vi "filter_bad_values.vi"(11 "Array 3":i16[](array[numeric])) -> (3 "Array 4":i32[](array[numeric]))   [LabVIEW 2012]
uses:
  <vilib>/NXT/Dual Mode Library/prims/addArrayElements_int.vi
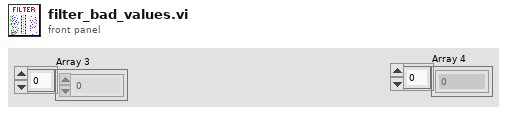
[diagram p1: front panel]
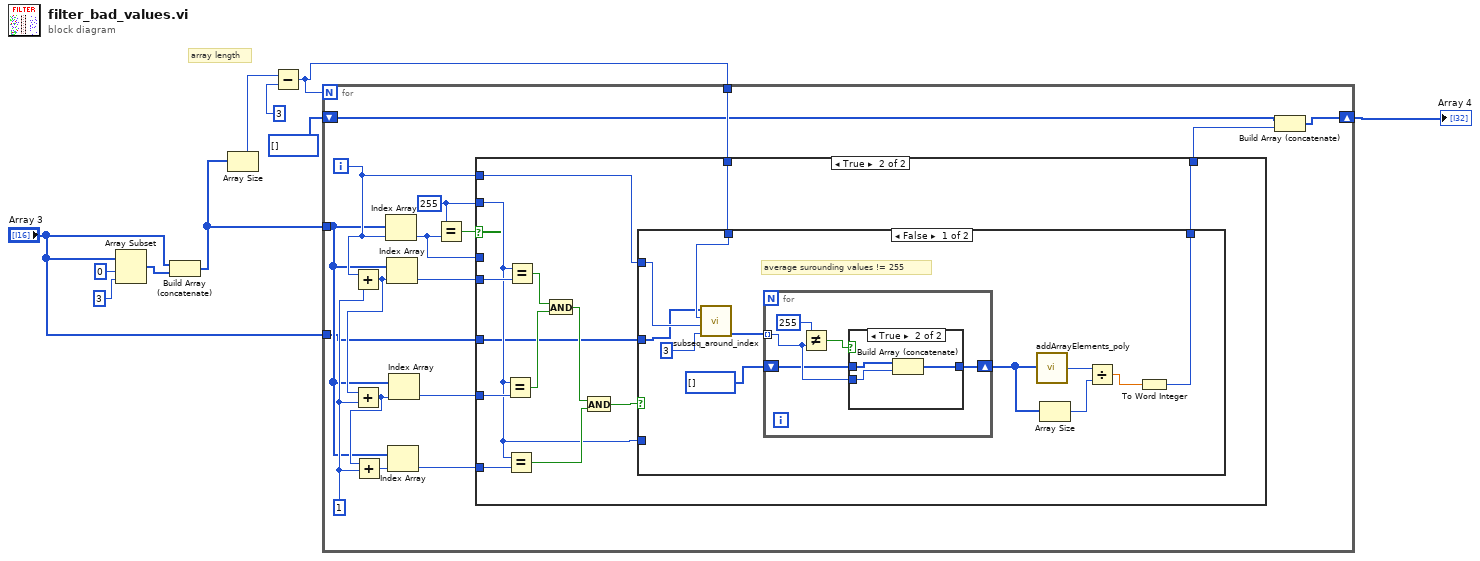
[diagram p0: block diagram]
diagram:
  # "array length"
  n1 = Array Subset(array="Array 3", index=0, length=3 ("index")) -> (w5:i16[])
  n2 = Build Array (concatenate)("Array 3", w5) -> (w4:i16[])
  n3 = Array Size(array=w4) -> (size(s)=w9:i32)
  n4 = Subtract(x=w9, y=3) -> (x-y=w2:i32)
  n5 = for {
    N: w2 -> [_]
    tunnel: w4 -> [w12]
    shift-right: [w13] -> w1
    shift-left: i32[] [] -> [w14]
    tunnel: w2 -> [w17]
    tunnel: "Array 3" -> [w11]
    i -> [w18]
    w19 = 255
    w26 = 1
    n6 = Add(x=w18, y=w26) -> (x+y=w25:i32)
    n7 = Add(x=w25, y=w26) -> (x+y=w24:i32)
    n8 = Add(x=w24, y=w26) -> (x+y=w27:i32)
    n9 = Index Array(array=w12, index=w18) -> (element=w16:i16)
    n10 = Index Array(array=w12, index=w25) -> (element=w22:i16)
    n11 = Index Array(array=w12, index=w27) -> (element=w20:i16)
    n12 = Index Array(array=w12, index=w24) -> (element=w21:i16)
    n13 = Equal?(x=w19, y=w16) -> (x = y?=w23:bool)
    n14 = case shown="True" w23 {
      tunnel: w22 -> [_ w39]
      tunnel: w21 -> [_ w40]
      tunnel: w20 -> [_ w41]
      tunnel: w19 -> [_ w33]
      tunnel: w18 -> [_ w32]
      tunnel: w17 -> [_ w31]
      tunnel: [w28 w30] -> w15
      tunnel: w16 -> [w28 _]
      tunnel: w11 -> [_ w29]
      frame False {
      }
      frame True {
        n15 = Equal?(x=w33, y=w40) -> (x = y?=w37:bool)
        n16 = Equal?(x=w33, y=w41) -> (x = y?=w35:bool)
        n17 = Equal?(x=w33, y=w39) -> (x = y?=w38:bool)
        n18 = And(x=w38, y=w37) -> (x .and. y?=w36:bool)
        n19 = And(x=w36, y=w35) -> (x .and. y?=w34:bool)
        n20 = case shown="False" w34 {
          tunnel: w33 -> [_ w62]
          tunnel: [w45 w62] -> w30
          tunnel: w32 -> [w52 _]
          tunnel: w31 -> [w51 _]
          tunnel: w29 -> [w42 _]
          frame False {
            # "average surounding values != 255"
            n21 = call "subseq_around_index.vi"("length around index 2"=3 ("length around index"), "index 2"=w52, "array length 2"=w51, "Array 3"=w42) -> ("Array 2"=w50:i32[])  [unwired: 7 in]
            n22 = for {
              tunnel: w50 -> [w55] mode=indexing
              shift-right: [w54] -> w47
              shift-left: i32[] [] -> [w53]
              n23 = Not Equal?(x=255 ("y"), y=w55) -> (x != y?=w57:bool)
              n24 = case shown="True" w57 {
                tunnel: w55 -> [_ w61]
                tunnel: [w58 w60] -> w54
                tunnel: w53 -> [w58 w59]
                frame False {
                }
                frame True {
                  n25 = Build Array (concatenate)(w59, w61) -> (w60:i32[])
                }
              }
            }
            n26 = call-poly <vilib>:"addArrayElements_poly.vi"("Numeric Array"=w47) -> ("Sum"=w49:i32)
            n27 = Array Size(array=w47) -> (size(s)=w48:i32)
            n28 = Divide(x=w49, y=w48) -> (x/y=w46:dbl)
            n29 = To Word Integer(number=w46) -> (16bit integer=w45:i16)
          }
          frame True {
            # "255"
          }
        }
      }
    }
    n30 = Build Array (concatenate)(w14, w15) -> (w13:i32[])
  }
  "Array 4" <- w1
